vi "VI Temp Path.vi"(11 "Extension (\"vi\")":string="vi") -> (3 "Path (.vi)":path)   [LabVIEW 2022 SP3, in "VI-Snippet.lvlib"]
doc: "Returns a temporary filename path with the <b>Extension</b> provided."
uses:
  VI-Snippet.lvlib
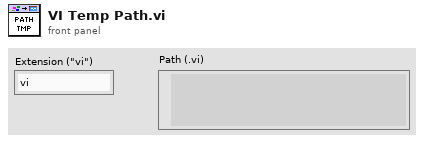
[diagram p1: front panel]
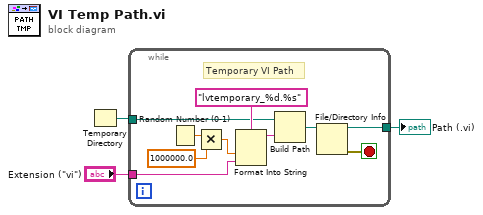
[diagram p0: block diagram]
diagram:
  n1 = Temporary Directory() -> (w1:path)
  n2 = while {
    tunnel: "Extension (\"vi\")" -> [w5]
    tunnel: [w6] -> w2
    tunnel: w1 -> [w4]
    stop <- w7 stop-if-true
    # "Temporary VI Path"
    n3 = Random Number (0-1)() -> (number: 0 to 1=w13:dbl)
    n4 = Multiply(x=w13, y=1000000.0) -> (x*y=w10:dbl)
    n5 = Format Into String(format string="lvtemporary_%d.%s", w10, w5) -> (resulting string=w9:string)  [unwired: 2 in, 1 out]
    n6 = Build Path(base path=w4, name or relative path=w9) -> (appended path=w8:path)
    n7 = File/Directory Info(path=w8) -> (path out=w6:path, error out=w7:errorcluster)  [unwired: 1 in, 5 out]
  }
  "Path (.vi)" <- w2
